vi "Configure Calc Compare.vi"(5 "Limit Lower (0)":dbl min=0.0 max=999999000000.0 step=1e-15 format="%_6g", 6 "Limit Upper (0)":dbl min=0.0 max=999999000000.0 step=1e-15 format="%_6g", 7 "error in (no error)":errorcluster, 9 "Calculate Comparator  (0: Off)":u16(ring) format="%_1g" items=["Off", "On"], 10 "VISA resource name":refnum<visa-resource-name>) -> (0 "error out":errorcluster, 3 "VISA resource name out":refnum<visa-resource-name>)   [LabVIEW 2017, in "ADCMT7451_ADC.lvlib"]
doc: "Enables or disables the comparator calculation."
uses:
  ADCMT7451_ADC.lvlib
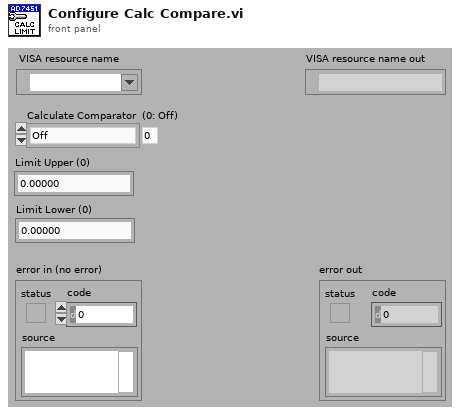
[diagram p1: front panel]
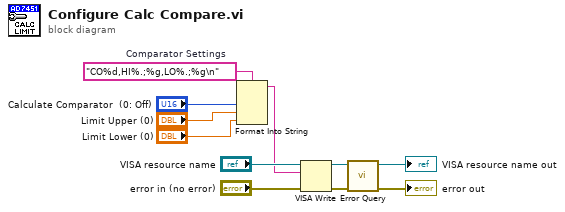
[diagram p0: block diagram]
diagram:
  w2 = "CO%d,HI%.;%g,LO%.;%g\n"  # Comparator Settings
  n1 = Format Into String(format string=w2, "Calculate Comparator  (0: Off)", "Limit Upper (0)", "Limit Lower (0)") -> (resulting string=w1:string)  [unwired: 2 in, 1 out]
  n2 = VISA Write(VISA resource name="VISA resource name", write buffer=w1, error in (no error)="error in (no error)") -> (VISA resource name out=w7:refnum<visa-resource-name>, error out=w6:errorcluster)  [unwired: 1 out]
  n3 = call "Error Query.vi"("error in (no error)"=w6, "VISA resource name"=w7) -> ("error out"=→"error out":errorcluster, "VISA resource name out"=→"VISA resource name out":refnum<visa-resource-name>)  [unwired: 6 in, 2 out]
